vi "Write Cuenta.vi"(10 "Cuenta":dbl, 11 "Hijo in":refnum<class "Hijo.lvclass">) -> (3 "Hijo out":refnum<class "Hijo.lvclass">)   [LabVIEW 2020, in "Hijo.lvlib" / "Hijo.lvclass"]
uses:
  Hijo.lvclass
  Hijo.lvclass/Hijo.ctl
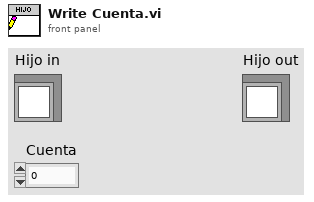
[diagram p1: front panel]
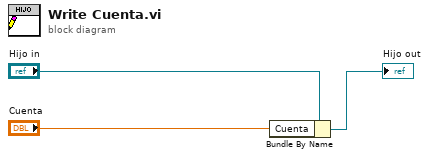
[diagram p0: block diagram]
diagram:
  n1 = Bundle By Name(cluster="Hijo in", "Cuenta"="Cuenta") -> (→"Hijo out":refnum<class "Hijo.lvclass">)
